vi "Test Empty String-Path.vi"(8 "error in (no error)":errorcluster) -> (0 "error out":errorcluster, 3 "Pass?":bool)   [LabVIEW 2020]
uses:
  G-Unicode/Types/UTF-8 Path/UTF-8 Path.lvclass
  G-Unicode/Types/UTF-8 Path/UTF-8 Path.lvclass/UTF-8 Path.ctl
  G-Unicode/Types/UTF-8 String/UTF-8 String.lvclass
  G-Unicode/Types/UTF-8 String/UTF-8 String.lvclass/UTF-8 String.ctl
  ad46b0ad-ad46-4f53-b267-1a4edb1f84ba.vi
  bc3c3682-5788-4fde-b95d-512f2fdda15d.vi
  697d9262-8cb1-4530-a1c3-7d4a6b35f797.vi
  cfb0af94-1a9a-40a2-9481-5d930b535457.vi
  418c229c-3535-4052-8df9-854bdd0df0df.vi
  1380012a-c389-4ab7-9e9f-faa4a8ccdd99.vi
  685bc419-866f-4371-a32c-8e0ee959b027.vi
  e91a8ab1-7c3a-455b-886b-e84049f193fe.vi
  G-Unicode/Private/Conversion/Text to UTF-8.vi
  G-Unicode/Private/Conversion/Polymorphic VIs/Text to UTF-8 (LabVIEW String).vi
  G-Unicode/Private/Conversion/Text as String.vi
  G-Unicode/Private/Conversion/Polymorphic VIs/Text as String (UTF-8 Path).vi
  G-Unicode/Private/Conversion/Polymorphic VIs/Text as String (LabVIEW Path).vi
  G-Unicode/Private/Conversion/Polymorphic VIs/Text as String (UTF-8 String).vi
  G-Unicode/Private/Conversion/Polymorphic VIs/Text as String (LabVIEW String).vi
  G-Unicode/Types/UTF-8 Path/Read Encoded UTF-8 Path.vi
  G-Unicode/Types/UTF-8 String/Read Encoded UTF-8 String.vi
  G-Unicode/Unicode/Detect String Encoding.vi
  G-Unicode/Private/Conversion/Encoded UTF-16LE String to Encoded UTF-8 String.vi
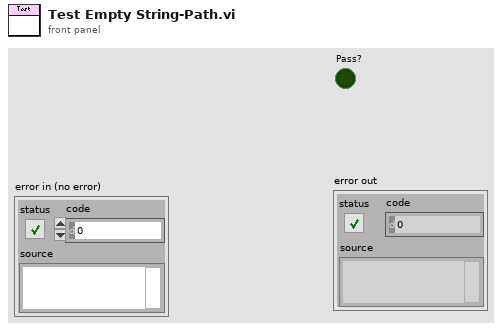
[diagram p1: front panel]
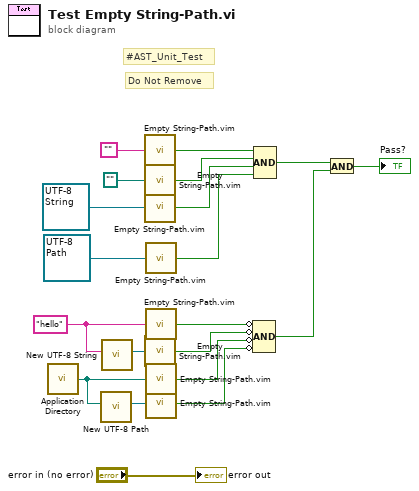
[diagram p0: block diagram]
diagram:
  w2 = "hello"
  # "Do Not Remove"
  # "#AST_Unit_Test"
  n1 = call <vilib>:"Application Directory.vi"() -> ("Application Directory"=w4:path)
  n2 = call "New UTF-8 Path.vi"("LabVIEW Path"=w4) -> ("UTF-8 Path"=w3:refnum<class "UTF-8 Path.lvclass">)  [unwired: 9 in, 1 out]
  n3 = call "New UTF-8 String.vi"("String"=w2) -> ("UTF-8 String"=w1:refnum<class "UTF-8 String.lvclass">)  [unwired: 9 in, 1 out]
  n4 = call "Empty String-Path.vim"("String/Path"="") -> ("Empty?"=w20:bool)
  n5 = call "Empty String-Path.vim"("String/Path"=path "") -> ("Empty?"=w17:bool)
  n6 = call "Empty String-Path.vim"("String/Path"=refnum<class "UTF-8 String.lvclass"> refnum ("G-Unicode.lvlib:UTF-8 String.lvclass")) -> ("Empty?"=w13:bool)
  n7 = call "Empty String-Path.vim"("String/Path"=w1) -> ("Empty?"=w5:bool)
  n8 = call "Empty String-Path.vim"("String/Path"=refnum<class "UTF-8 Path.lvclass"> refnum ("G-Unicode.lvlib:UTF-8 Path.lvclass")) -> ("Empty?"=w12:bool)
  n9 = call "Empty String-Path.vim"("String/Path"=w2) -> ("Empty?"=w6:bool)
  n10 = call "Empty String-Path.vim"("String/Path"=w4) -> ("Empty?"=w8:bool)
  n11 = call "Empty String-Path.vim"("String/Path"=w3) -> ("Empty?"=w7:bool)
  n12 = Compound Arithmetic op=AND(invert w6, invert w5, invert w8, invert w7) -> (w9:bool)
  n13 = Compound Arithmetic op=AND(w20, w17, w13, w12) -> (w11:bool)
  n14 = And(x=w11, y=w9) -> (x .and. y?=→"Pass?":bool)
  "error out" <- "error in (no error)"
